vi "StandAloneTransient_NIDCPOWER_PSU_POWER_OFF_V1.vi"(8 "error in":errorcluster caption="error in (no error)", 10 "channel name":string, 11 "resource name":refnum<k15>="PS_4110" caption="Hardware Force Reset") -> (0 "eRROR OUT":errorcluster caption="error out")   [LabVIEW 2019]
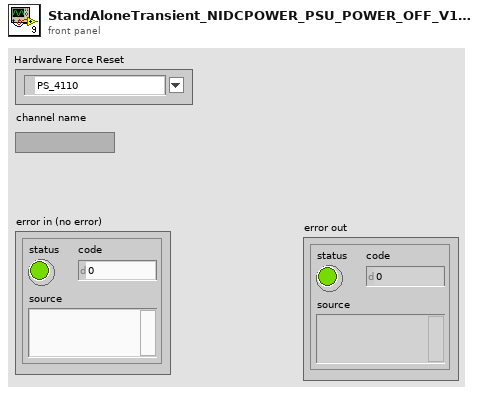
[diagram p1: front panel]
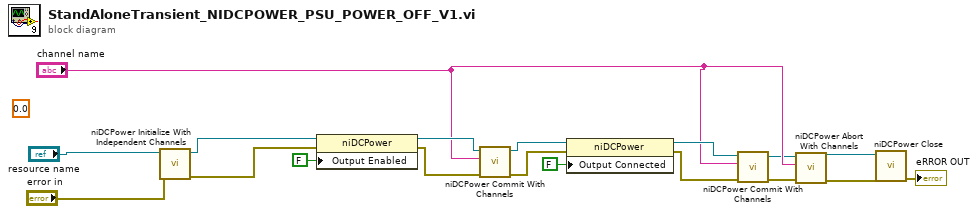
[diagram p0: block diagram]
diagram:
  (unwired) 0.0 ("voltage level")
  n1 = call <instrlib>:"niDCPower Initialize With Independent Channels.vi"("error in (no error)"="error in", "resource name"="resource name") -> ("error out"=w15:errorcluster, "instrument handle out"=w14:refnum<k15>)  [unwired: 8 in]
  n2 = property class="niDCPower"(reference=w14, error in=w15, "Output Enabled"=FALSE ("Source:Output Enabled")) -> (reference out=w9:refnum<k15>, error out=w8:errorcluster)
  n3 = call <instrlib>:"niDCPower Commit With Channels.vi"("error in (no error)"=w8, "channel name"="channel name", "instrument handle"=w9) -> ("error out"=w6:errorcluster, "instrument handle out"=w7:refnum<k15>)  [unwired: 7 in]
  n4 = property class="niDCPower"(reference=w7, error in=w6, "Output Connected"=FALSE ("Source:Output Connected")) -> (reference out=w5:refnum<k15>, error out=w4:errorcluster)
  n5 = call <instrlib>:"niDCPower Commit With Channels.vi"("error in (no error)"=w4, "channel name"="channel name", "instrument handle"=w5) -> ("error out"=w1:errorcluster, "instrument handle out"=w2:refnum<k15>)  [unwired: 7 in]
  n6 = call <instrlib>:"niDCPower Abort With Channels.vi"("error in (no error)"=w1, "channel name"="channel name", "instrument handle"=w2) -> ("error out"=w11:errorcluster, "instrument handle out"=w12:refnum<k15>)  [unwired: 7 in]
  n7 = call <instrlib>:"niDCPower Close.vi"("error in (no error)"=w11, "instrument handle"=w12) -> ("error out"=→"eRROR OUT":errorcluster)  [unwired: 9 in]
